vi "forumlate message write.vi"(9 "can?":bool, 10 "SpyMessage{}":T1={"StatusBitField"=0, "StatusBitField2"=0, "TimeHardware"=0, "TimeHardware2"=0, "TimeSystem"=0, "TimeSystem2"=0, "TimeStampHardwareID"=0, "TimeStampHardwareID2"=0, "NetworkID"=0, "NodeID"=0, "Protocol"=0, "MessagePieceID"=0, "ColorID"=0, "NumberBytesHeader"=0, "NumberBytesData"=0, "DescriptionID"=0, "ArbIDOrHeader"=0, "Data [8]"=[0, 0, 0, 0, 0, 0, 0, 0], "AckBytes [8]"=[0, 0, 0, 0, 0, 0, 0, 0], "Value"=0.0, "MiscData"=0} {"AckBytes [8]" format="%.0x"; "Data [8]" format="%.0x"; "ArbIDOrHeader" format="%.0x"; "DescriptionID" format="%.0x"; "NetworkID" format="%.0x"}) -> (2 "Messages Raw OUT":u8[](array[numeric]) format="%.0x")   [LabVIEW 2009]
uses:
  ctl spymessage.ctl
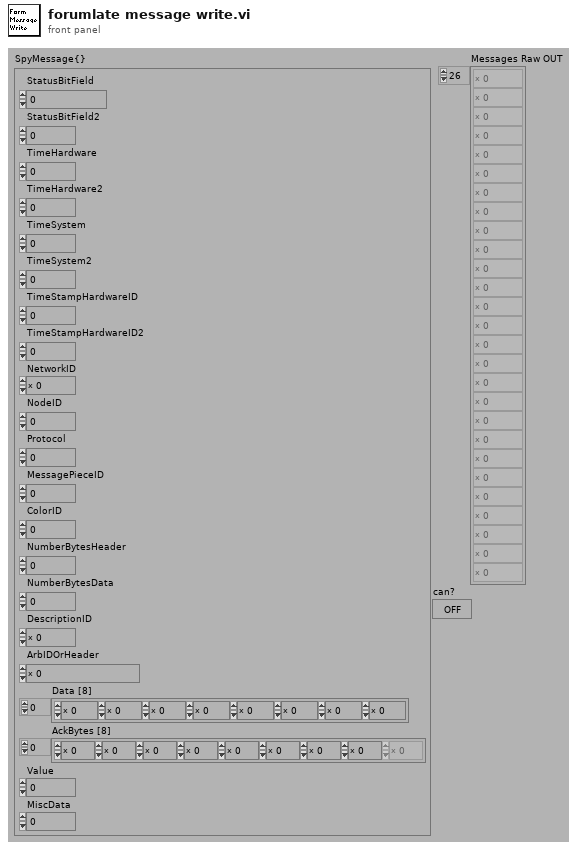
[diagram p1: front panel]
types:
  T1 = typedef "ctl spymessage.ctl" = cluster{"StatusBitField":u32, "StatusBitField2":u32, "TimeHardware":u32, "TimeHardware2":u32, "TimeSystem":u32, "TimeSystem2":u32, "TimeStampHardwareID":u8, "TimeStampHardwareID2":u8, "NetworkID":u8, "NodeID":u8, "Protocol":u8, "MessagePieceID":u8, "ColorID":u8, "NumberBytesHeader":u8, "NumberBytesData":u8, "DescriptionID":u16, "ArbIDOrHeader":u32, "Data [8]":u8[], "AckBytes [8]":u8[], "Value":sgl, "MiscData":u8}
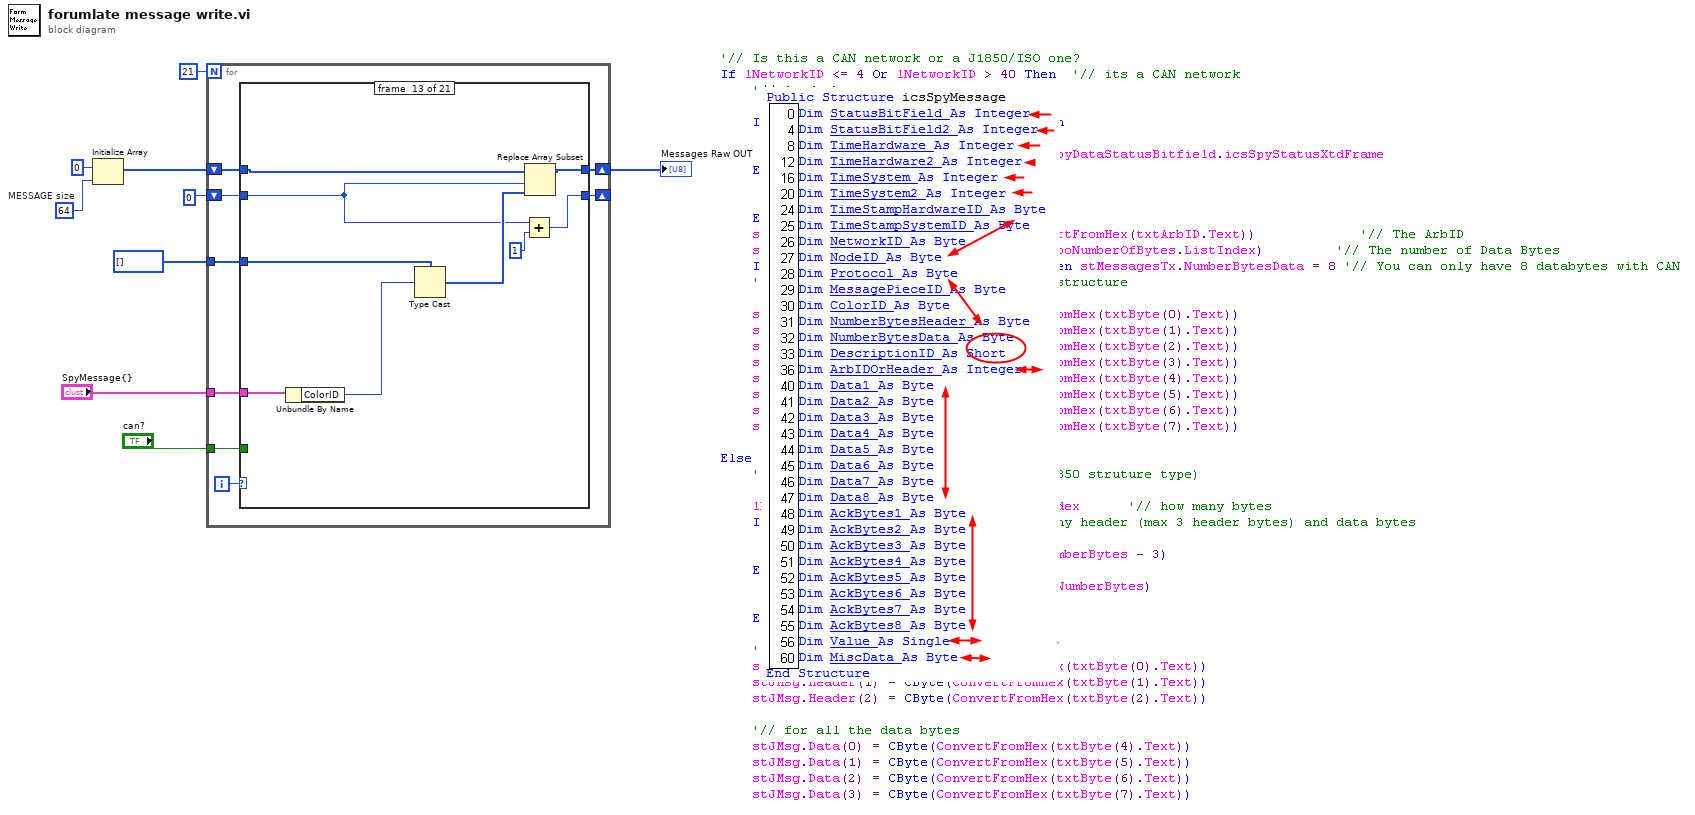
[diagram p0: block diagram]
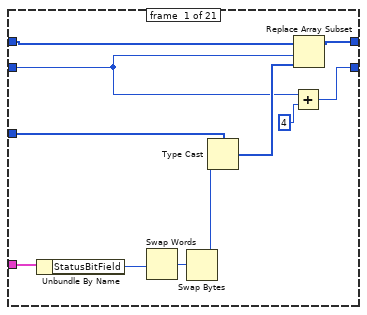
[diagram p2: hidden frame]
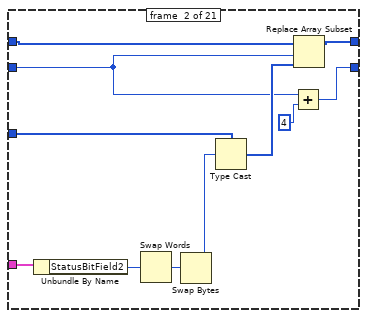
[diagram p3: hidden frame]
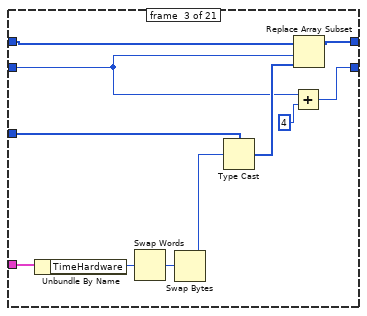
[diagram p4: hidden frame]
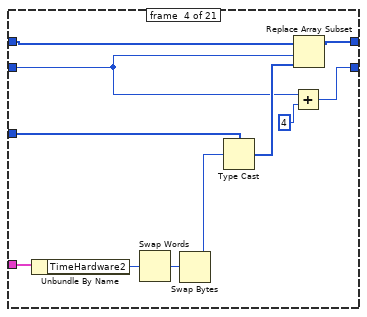
[diagram p5: hidden frame]
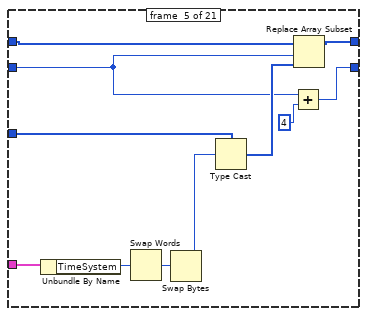
[diagram p6: hidden frame]
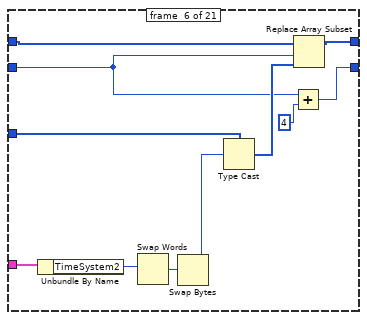
[diagram p7: hidden frame]
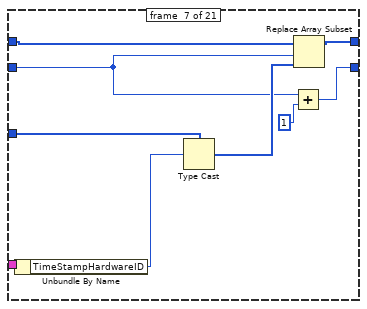
[diagram p8: hidden frame]
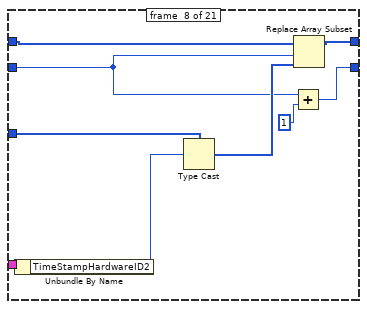
[diagram p9: hidden frame]
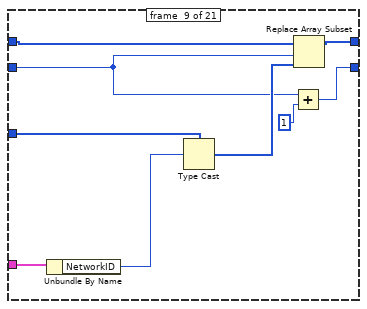
[diagram p10: hidden frame]
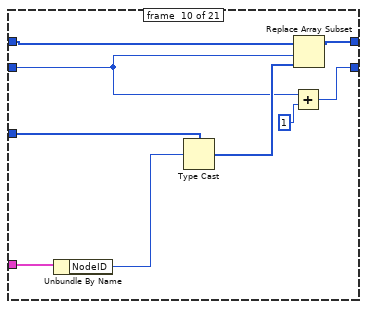
[diagram p11: hidden frame]
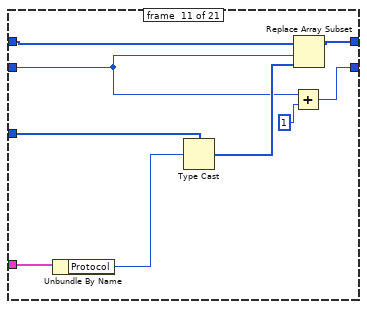
[diagram p12: hidden frame]
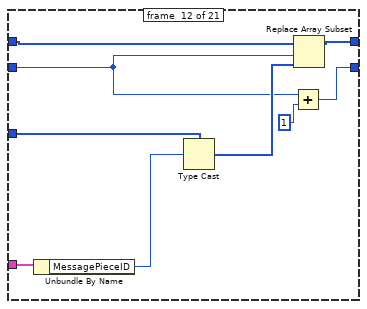
[diagram p13: hidden frame]
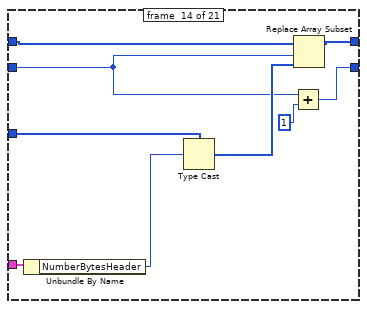
[diagram p14: hidden frame]
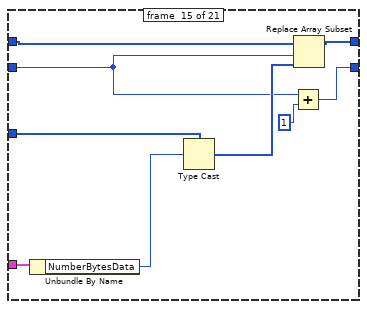
[diagram p15: hidden frame]
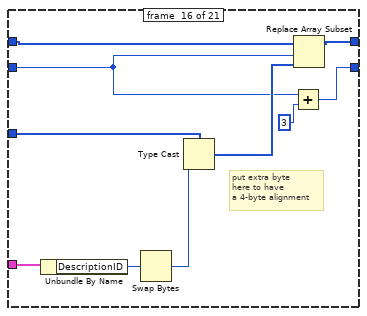
[diagram p16: hidden frame]
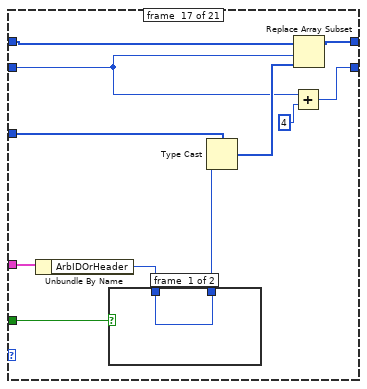
[diagram p17: hidden frame]
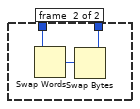
[diagram p18: hidden frame]
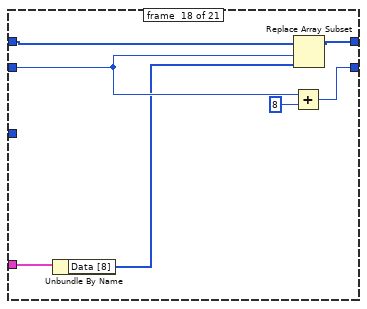
[diagram p19: hidden frame]
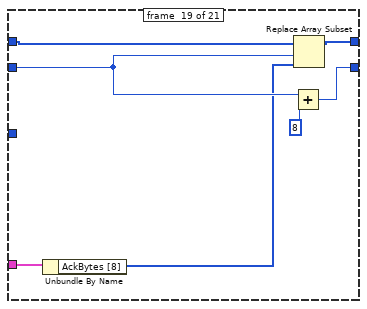
[diagram p20: hidden frame]
diagram:
  w6 = 64  # MESSAGE size
  n1 = Initialize Array(u8 0 ("element"), w6) -> (w5:u8[])
  n2 = for {
    N: 21 -> [_]
    tunnel: "SpyMessage{}" -> [w16]
    shift-right: [w11] -> w2
    shift-left: w5 -> [w15]
    tunnel: u8[] [] ("initialized array") -> [w14]
    shift-right: [w12] -> _
    shift-left: 0 ("element") -> [w13]
    tunnel: "can?" -> [w10]
    i -> [w17]
    n3 = case shown="16" w17 {
      tunnel: w16 -> [w28 w39 w50 w61 w72 w83 w92 w101 w110 w119 w128 w137 w146 w155 w164 w174 w185 w196 w203 w212 w221]
      tunnel: w15 -> [w27 w38 w49 w60 w71 w82 w91 w100 w109 w118 w127 w136 w145 w154 w163 w173 w184 w195 w202 w211 w220]
      tunnel: w14 -> [w26 w37 w48 w59 w70 w81 w89 w98 w107 w116 w125 w134 w143 w152 w161 w172 w183 _ _ w209 w218]
      tunnel: w13 -> [w24 w35 w46 w57 w68 w79 w87 w96 w105 w114 w123 w132 w141 w150 w159 w170 w181 w194 w201 w207 w216]
      tunnel: [w22 w33 w44 w55 w66 w77 w85 w94 w103 w112 w121 w130 w139 w148 w157 w168 w179 w193 w200 w205 w214] -> w12
      tunnel: [w21 w32 w43 w54 w65 w76 w84 w93 w102 w111 w120 w129 w138 w147 w156 w167 w178 w192 w199 w204 w213] -> w11
      tunnel: w10 -> [_ _ _ _ _ _ _ _ _ _ _ _ _ _ _ _ w175 _ _ _ _]
      frame #0 {
        n4 = Unbundle By Name(w28) -> ("StatusBitField"=w19:u32)
        n5 = Swap Words(1:w19) -> (0:w20:u32)
        n6 = Swap Bytes(anything=w20) -> (byte swapped=w18:u32)
        n7 = Type Cast(type=w26, x=w18) -> (*(type *) &x=w25:u8[])
        n8 = Add(x=w24, y=4) -> (x+y=w22:i32)
        n9 = Replace Array Subset(array=w27, new element=w25, index=w24) -> (w21:u8[])
      }
      frame #1 {
        n10 = Unbundle By Name(w39) -> ("StatusBitField2"=w30:u32)
        n11 = Swap Words(1:w30) -> (0:w31:u32)
        n12 = Swap Bytes(anything=w31) -> (byte swapped=w29:u32)
        n13 = Type Cast(type=w37, x=w29) -> (*(type *) &x=w36:u8[])
        n14 = Add(x=w35, y=4) -> (x+y=w33:i32)
        n15 = Replace Array Subset(array=w38, new element=w36, index=w35) -> (w32:u8[])
      }
      frame #2 {
        n16 = Unbundle By Name(w50) -> ("TimeHardware"=w41:u32)
        n17 = Swap Words(1:w41) -> (0:w42:u32)
        n18 = Swap Bytes(anything=w42) -> (byte swapped=w40:u32)
        n19 = Type Cast(type=w48, x=w40) -> (*(type *) &x=w47:u8[])
        n20 = Add(x=w46, y=4) -> (x+y=w44:i32)
        n21 = Replace Array Subset(array=w49, new element=w47, index=w46) -> (w43:u8[])
      }
      frame #3 {
        n22 = Unbundle By Name(w61) -> ("TimeHardware2"=w52:u32)
        n23 = Swap Words(1:w52) -> (0:w53:u32)
        n24 = Swap Bytes(anything=w53) -> (byte swapped=w51:u32)
        n25 = Type Cast(type=w59, x=w51) -> (*(type *) &x=w58:u8[])
        n26 = Add(x=w57, y=4) -> (x+y=w55:i32)
        n27 = Replace Array Subset(array=w60, new element=w58, index=w57) -> (w54:u8[])
      }
      frame #4 {
        n28 = Unbundle By Name(w72) -> ("TimeSystem"=w63:u32)
        n29 = Swap Words(1:w63) -> (0:w64:u32)
        n30 = Swap Bytes(anything=w64) -> (byte swapped=w62:u32)
        n31 = Type Cast(type=w70, x=w62) -> (*(type *) &x=w69:u8[])
        n32 = Add(x=w68, y=4) -> (x+y=w66:i32)
        n33 = Replace Array Subset(array=w71, new element=w69, index=w68) -> (w65:u8[])
      }
      frame #5 {
        n34 = Unbundle By Name(w83) -> ("TimeSystem2"=w74:u32)
        n35 = Swap Words(1:w74) -> (0:w75:u32)
        n36 = Swap Bytes(anything=w75) -> (byte swapped=w73:u32)
        n37 = Type Cast(type=w81, x=w73) -> (*(type *) &x=w80:u8[])
        n38 = Add(x=w79, y=4) -> (x+y=w77:i32)
        n39 = Replace Array Subset(array=w82, new element=w80, index=w79) -> (w76:u8[])
      }
      frame #6 {
        n40 = Unbundle By Name(w92) -> ("TimeStampHardwareID"=w90:u8)
        n41 = Type Cast(type=w89, x=w90) -> (*(type *) &x=w88:u8[])
        n42 = Add(x=w87, y=1) -> (x+y=w85:i32)
        n43 = Replace Array Subset(array=w91, new element=w88, index=w87) -> (w84:u8[])
      }
      frame #7 {
        n44 = Unbundle By Name(w101) -> ("TimeStampHardwareID2"=w99:u8)
        n45 = Type Cast(type=w98, x=w99) -> (*(type *) &x=w97:u8[])
        n46 = Add(x=w96, y=1) -> (x+y=w94:i32)
        n47 = Replace Array Subset(array=w100, new element=w97, index=w96) -> (w93:u8[])
      }
      frame #8 {
        n48 = Unbundle By Name(w110) -> ("NetworkID"=w108:u8)
        n49 = Type Cast(type=w107, x=w108) -> (*(type *) &x=w106:u8[])
        n50 = Add(x=w105, y=1) -> (x+y=w103:i32)
        n51 = Replace Array Subset(array=w109, new element=w106, index=w105) -> (w102:u8[])
      }
      frame #9 {
        n52 = Unbundle By Name(w119) -> ("NodeID"=w117:u8)
        n53 = Type Cast(type=w116, x=w117) -> (*(type *) &x=w115:u8[])
        n54 = Add(x=w114, y=1) -> (x+y=w112:i32)
        n55 = Replace Array Subset(array=w118, new element=w115, index=w114) -> (w111:u8[])
      }
      frame #10 {
        n56 = Unbundle By Name(w128) -> ("Protocol"=w126:u8)
        n57 = Type Cast(type=w125, x=w126) -> (*(type *) &x=w124:u8[])
        n58 = Add(x=w123, y=1) -> (x+y=w121:i32)
        n59 = Replace Array Subset(array=w127, new element=w124, index=w123) -> (w120:u8[])
      }
      frame #11 {
        n60 = Unbundle By Name(w137) -> ("MessagePieceID"=w135:u8)
        n61 = Type Cast(type=w134, x=w135) -> (*(type *) &x=w133:u8[])
        n62 = Add(x=w132, y=1) -> (x+y=w130:i32)
        n63 = Replace Array Subset(array=w136, new element=w133, index=w132) -> (w129:u8[])
      }
      frame #12 {
        n64 = Unbundle By Name(w146) -> ("ColorID"=w144:u8)
        n65 = Type Cast(type=w143, x=w144) -> (*(type *) &x=w142:u8[])
        n66 = Add(x=w141, y=1) -> (x+y=w139:i32)
        n67 = Replace Array Subset(array=w145, new element=w142, index=w141) -> (w138:u8[])
      }
      frame #13 {
        n68 = Unbundle By Name(w155) -> ("NumberBytesHeader"=w153:u8)
        n69 = Type Cast(type=w152, x=w153) -> (*(type *) &x=w151:u8[])
        n70 = Add(x=w150, y=1) -> (x+y=w148:i32)
        n71 = Replace Array Subset(array=w154, new element=w151, index=w150) -> (w147:u8[])
      }
      frame #14 {
        n72 = Unbundle By Name(w164) -> ("NumberBytesData"=w162:u8)
        n73 = Type Cast(type=w161, x=w162) -> (*(type *) &x=w160:u8[])
        n74 = Add(x=w159, y=1) -> (x+y=w157:i32)
        n75 = Replace Array Subset(array=w163, new element=w160, index=w159) -> (w156:u8[])
      }
      frame #15 {
        # "put extra byte\nhere to have\na 4-byte alignment"
        n76 = Unbundle By Name(w174) -> ("DescriptionID"=w166:u16)
        n77 = Swap Bytes(anything=w166) -> (byte swapped=w165:u16)
        n78 = Type Cast(type=w172, x=w165) -> (*(type *) &x=w171:u8[])
        n79 = Add(x=w170, y=3) -> (x+y=w168:i32)
        n80 = Replace Array Subset(array=w173, new element=w171, index=w170) -> (w167:u8[])
      }
      frame #16 {
        n81 = Unbundle By Name(w185) -> ("ArbIDOrHeader"=w177:u32)
        n82 = case shown="False" w175 {
          tunnel: w177 -> [w186 w188]
          tunnel: [w186 w187] -> w176
          frame #0 {
          }
          frame #1 {
            n83 = Swap Words(1:w188) -> (0:w189:u32)
            n84 = Swap Bytes(anything=w189) -> (byte swapped=w187:u32)
          }
        }
        n85 = Type Cast(type=w183, x=w176) -> (*(type *) &x=w182:u8[])
        n86 = Add(x=w181, y=4) -> (x+y=w179:i32)
        n87 = Replace Array Subset(array=w184, new element=w182, index=w181) -> (w178:u8[])
      }
      frame #17 {
        n88 = Unbundle By Name(w196) -> ("Data [8]"=w191:u8[])
        n89 = Add(x=w194, y=8) -> (x+y=w193:i32)
        n90 = Replace Array Subset(array=w195, new element=w191, index=w194) -> (w192:u8[])
      }
      frame #18 {
        n91 = Unbundle By Name(w203) -> ("AckBytes [8]"=w198:u8[])
        n92 = Add(x=w201, y=8) -> (x+y=w200:i32)
        n93 = Replace Array Subset(array=w202, new element=w198, index=w201) -> (w199:u8[])
      }
      frame #19 {
        n94 = Unbundle By Name(w212) -> ("Value"=w210:sgl)
        n95 = Type Cast(type=w209, x=w210) -> (*(type *) &x=w208:u8[])
        n96 = Add(x=w207, y=4) -> (x+y=w205:i32)
        n97 = Replace Array Subset(array=w211, new element=w208, index=w207) -> (w204:u8[])
      }
      frame #20 {
        n98 = Unbundle By Name(w221) -> ("MiscData"=w219:u8)
        n99 = Type Cast(type=w218, x=w219) -> (*(type *) &x=w217:u8[])
        n100 = Add(x=w216, y=1) -> (x+y=w214:i32)
        n101 = Replace Array Subset(array=w220, new element=w217, index=w216) -> (w213:u8[])
      }
    }
  }
  "Messages Raw OUT" <- w2
